vi "cDAQ DDS Close.vi"(8 "error in":errorcluster, 11 "cdaq session in":T1={"device"="", "channels"=[], "mclk source"="", "mclk [Hz]"=0.0, "fs [Hz]"=0.0, "block [s]"=0.0, "buf [s]"=0.0, "task"="", "cmd queue"=refnum, "proc ref"=refnum, "smpl clock out"="/cDAQ3/PFI0", "export smpl clock"=FALSE, "DC ofs [V]"=[], "timebase source"="", "timebase mode"=enum."Local"} {"channels" min=0 step=1}) -> (0 "error out":errorcluster, 3 "cdaq session out":T1={"device"="", "channels"=[], "mclk source"="", "mclk [Hz]"=0.0, "fs [Hz]"=0.0, "block [s]"=0.0, "buf [s]"=0.0, "task"="", "cmd queue"=refnum, "proc ref"=refnum, "smpl clock out"="/cDAQ3/PFI0", "export smpl clock"=FALSE, "DC ofs [V]"=[], "timebase source"="", "timebase mode"=enum."Local"} {"channels" min=0 step=1})   [LabVIEW 2020]
uses:
  cDAQ DDS Session.ctl
  cDAQ DDS Setup.ctl
  cDAQ DDS Timebase Mode.ctl
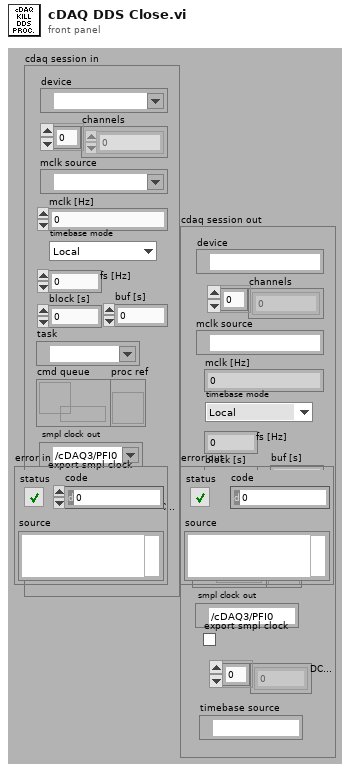
[diagram p1: front panel]
types:
  T1 = typedef "cDAQ DDS Session.ctl" = cluster{"device":tag, "channels":i32[], "mclk source":tag, "mclk [Hz]":dbl, "fs [Hz]":dbl, "block [s]":dbl, "buf [s]":dbl, "task":refnum<k21>, "cmd queue":refnum<queue>, "proc ref":refnum<vi>, "smpl clock out":tag, "export smpl clock":bool, "DC ofs [V]":dbl[], "timebase source":tag, "timebase mode":T2}
  T2 = typedef "cDAQ DDS Timebase Mode.ctl" = enum16{"Local", "Take from ADC (e.g. NI 9238)", "Other source"}
  T3 = typedef "cDAQ DDS Setup.ctl" = cluster{"A [V]":dbl[], "ph [rad]":dbl[], "f [Hz]":dbl[], "stop":bool, "ofs [V]":dbl[]}
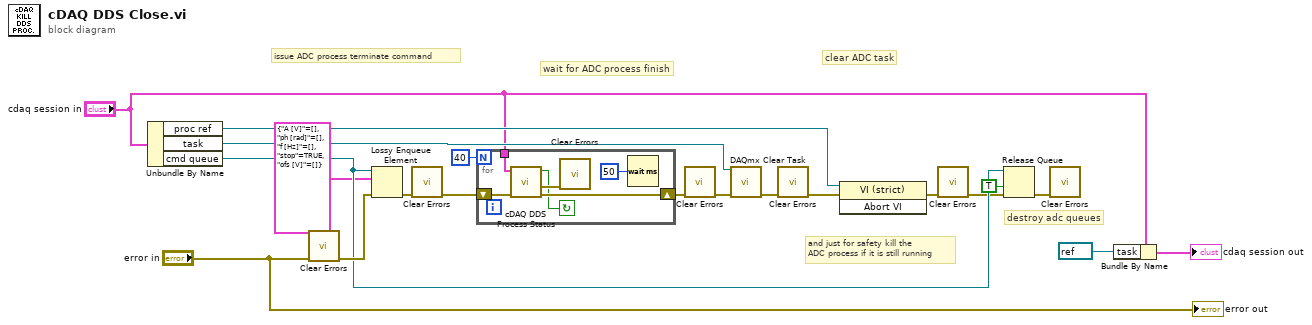
[diagram p0: block diagram]
diagram:
  # "destroy adc queues"
  # "and just for safety kill the\nADC process if it is still running"
  # "clear ADC task"
  # "wait for ADC process finish"
  # "issue ADC process terminate command"
  n1 = Unbundle By Name("cdaq session in") -> ("proc ref"=w11:refnum<vi>, "task"=w13:refnum<k21>, "cmd queue"=w9:refnum<queue>)
  n2 = call <vilib>:"Clear Errors.vi"("error in (no error)"="error in") -> ("error out"=w12:errorcluster)  [unwired: 5 in, 1 out]
  n3 = Lossy Enqueue Element(queue=w9, element=T3 {"A [V]"=[], "ph [rad]"=[], "f [Hz]"=[], "stop"=TRUE, "ofs [V]"=[]}, error in (no error)=w12) -> (error out=w18:errorcluster)  [unwired: 3 out]
  n4 = call <vilib>:"Clear Errors.vi"("error in (no error)"=w18) -> ("error out"=w17:errorcluster)  [unwired: 5 in, 1 out]
  n5 = for {
    N: 40 -> [_]
    shift-right: [w25] -> w15
    shift-left: w17 -> [w26]
    tunnel: "cdaq session in" -> [w21]
    stop <- w23 continue-if-true
    n6 = call "cDAQ DDS Process Status.vi"("error in"=w26, "cDAQ dds"=w21) -> ("error out"=w25:errorcluster, "sweep error out"=w24:errorcluster, "is running"=w23:bool)  [unwired: 7 in]
    n7 = call <vilib>:"Clear Errors.vi"("error in (no error)"=w24) -> ()  [unwired: 5 in, 2 out]
    n8 = Wait (ms)(milliseconds to wait=u32 50) -> ()  [unwired: 1 out]
  }
  n9 = call <vilib>:"Clear Errors.vi"("error in (no error)"=w15) -> ("error out"=w14:errorcluster)  [unwired: 5 in, 1 out]
  n10 = call <vilib>:"DAQmx Clear Task.vi"("task in"=w13, "error in"=w14) -> ("error out"=w10:errorcluster)  [unwired: 13 in]
  n11 = call <vilib>:"Clear Errors.vi"("error in (no error)"=w10) -> ("error out"=w2:errorcluster)  [unwired: 5 in, 1 out]
  n12 = invoke class="VI (strict)" method="Abort VI"(reference=w11, error in=w2) -> (error out=w7:errorcluster)  [unwired: 1 in, 2 out]
  n13 = call <vilib>:"Clear Errors.vi"("error in (no error)"=w7) -> ("error out"=w6:errorcluster)  [unwired: 5 in, 1 out]
  n14 = Release Queue(queue=w9, force destroy? (F)=TRUE, error in (no error)=w6) -> (error out=w3:errorcluster)  [unwired: 2 out]
  n15 = call <vilib>:"Clear Errors.vi"("error in (no error)"=w3) -> ()  [unwired: 5 in, 2 out]
  n16 = Bundle By Name(cluster="cdaq session in", "task"=refnum<k21> refnum ("ADC task")) -> (→"cdaq session out":T1)
  "error out" <- "error in"
